vi "TapeComponents.vi"() -> ()   [LabVIEW 2021]
panel:
  in  "OperationsPos2":cluster{"GoToBP":bool, "DropTool":bool}={"GoToBP"=TRUE, "DropTool"=TRUE}
  in  "VacuumStates":path=path "C:/Users/TTUHEP/Documents/LabVIEW/GantryPrograms/Configs/TapeCompPickPlaceVacuumStates.json"
  in  "GoHome":bool
  in  "OperationsPos1":T1={"GoToToolPos"=TRUE, "PickTool"=TRUE, "GoToSenPCB"=TRUE, "PickSiPCB"=TRUE}
  out "Error Out":errorcluster
  in  "Error In":errorcluster
  in  "Zone":enum16{"ZoneA", "ZoneB", "ZoneC", "ZoneD"}(ring)
  in  "AssmbType":enum16{"Sensor", "HB"}(ring)=enum."HB"
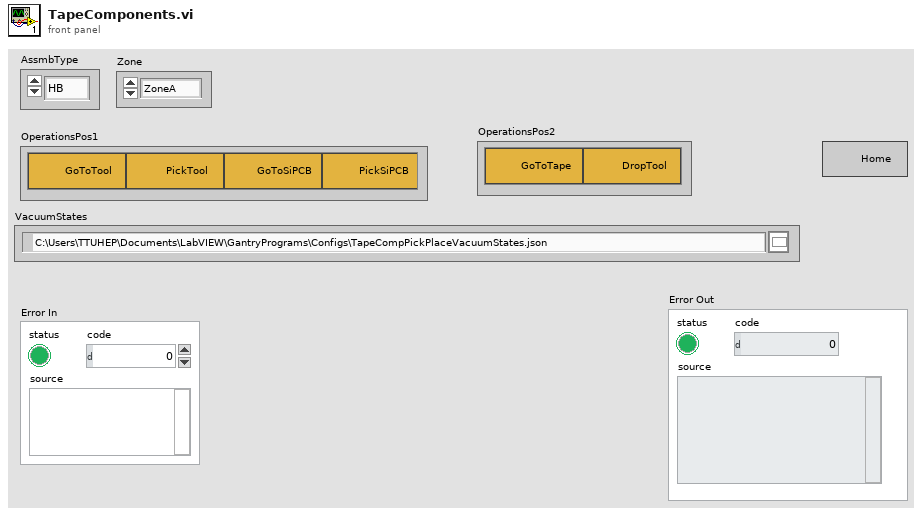
[diagram p1: front panel]
types:
  T1 = cluster{"GoToToolPos":bool, "PickTool":bool, "GoToSenPCB":bool, "PickSiPCB":bool}
  T2 = cluster{"[0]":bool, "[1]":bool, "[2]":bool, "[3]":bool, "[4]":bool, "[5]":bool}
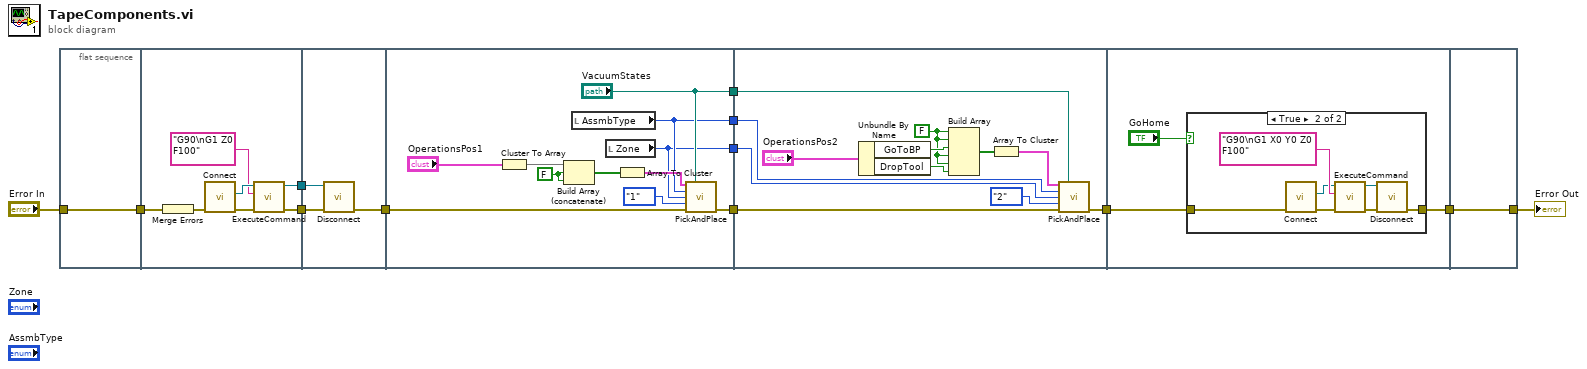
[diagram p0: block diagram]
diagram:
  n1 = flat-sequence {
    tunnel: [w13] -> w11
    tunnel: "Error In" -> [w13]
    tunnel: w11 -> [w14]
    tunnel: [w16] -> w10
    tunnel: [w15] -> w9
    tunnel: [w23] -> w8
    tunnel: w10 -> [w22]
    tunnel: w9 -> [w21]
    tunnel: w8 -> [w34]
    tunnel: [w33] -> w5
    tunnel: ["VacuumStates"] -> w3
    tunnel: [w25] -> w2
    tunnel: [w24] -> w1
    tunnel: w5 -> [w44]
    tunnel: [w39] -> w4
    tunnel: w3 -> [w45]
    tunnel: w2 -> [w41]
    tunnel: w1 -> [w40]
    tunnel: [w48] -> w12
    tunnel: w4 -> [w47]
    tunnel: w12 -> [w58]
    tunnel: [w58] -> w6
    frame #0 {
    }
    frame #1 {
      n2 = Merge Errors(w14) -> (w20:errorcluster)
      n3 = call "Connect.vi"("error in (no error)"=w20) -> ("error out"=w18:errorcluster, "controller"=w19:refnum<k24>)  [unwired: 9 in]
      n4 = call "ExecuteCommand.vi"("error in (no error)"=w18, "Command Code"="G90\nG1 Z0 F100", "controller in"=w19) -> ("error out"=w16:errorcluster, "controller out"=w15:refnum<k24>)  [unwired: 6 in, 1 out]
    }
    frame #2 {
      n5 = call "Disconnect.vi"("error in (no error)"=w22, "controller"=w21) -> ("error out"=w23:errorcluster)  [unwired: 9 in]
    }
    frame #3 {
      w28 = FALSE
      n6 = Cluster To Array(cluster="OperationsPos1") -> (array=w30:bool[])
      n7 = Build Array (concatenate)(w30, w28, w28) -> (w31:bool[])
      n8 = local read "AssmbType"() -> (w25:enum16{"Sensor", "HB"})
      n9 = local read "Zone"() -> (w24:enum16{"ZoneA", "ZoneB", "ZoneC", "ZoneD"})
      n10 = Array To Cluster(array=w31) -> (cluster=w27:T2)
      n11 = call "PickAndPlace.vi"("Operations"=w27, "VacuumStates"="VacuumStates", "AssmbType"=w25, "Zone"=w24, "Position"=enum16{"1", "2"}."1", "Error In"=w34) -> ("Error Out"=w33:errorcluster)  [unwired: 8 in, 1 out]
    }
    frame #4 {
      w36 = FALSE
      n12 = Unbundle By Name("OperationsPos2") -> ("GoToBP"=w37:bool, "DropTool"=w35:bool)
      n13 = Build Array(w36, w36, w37, w36, w36, w35) -> (w43:bool[])
      n14 = Array To Cluster(array=w43) -> (cluster=w42:T2)
      n15 = call "PickAndPlace.vi"("Operations"=w42, "VacuumStates"=w45, "AssmbType"=w41, "Zone"=w40, "Position"=enum16{"1", "2"}."2", "Error In"=w44) -> ("Error Out"=w39:errorcluster)  [unwired: 8 in, 1 out]
    }
    frame #5 {
      n16 = case shown="True" "GoHome" {
        tunnel: [w50 w51] -> w48
        tunnel: w47 -> [w50 w52]
        frame False {
        }
        frame True {
          n17 = call "Connect.vi"("error in (no error)"=w52) -> ("error out"=w57:errorcluster, "controller"=w54:refnum<k24>)  [unwired: 9 in]
          n18 = call "ExecuteCommand.vi"("error in (no error)"=w57, "Command Code"="G90\nG1 X0 Y0 Z0 F100", "controller in"=w54) -> ("error out"=w56:errorcluster, "controller out"=w53:refnum<k24>)  [unwired: 6 in, 1 out]
          n19 = call "Disconnect.vi"("error in (no error)"=w56, "controller"=w53) -> ("error out"=w51:errorcluster)  [unwired: 9 in]
        }
      }
    }
    frame #6 {
    }
  }
  "Error Out" <- w6
